vi "Error Lookup.vi"(8 "error in (no error)":errorcluster, 10 "Error code":i32, 11 "VISA resource name":refnum<visa-resource-name>) -> (0 "error out":errorcluster, 2 "Error Message":string, 3 "VISA resource name out":refnum<visa-resource-name>)   [LabVIEW 2012, in "Fluke 8508.lvlib"]
doc: "This utility VI references an instrument error code and returns the corresponding error description message."
uses:
  Fluke 8508.lvlib
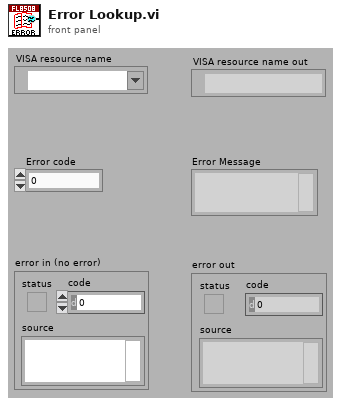
[diagram p1: front panel]
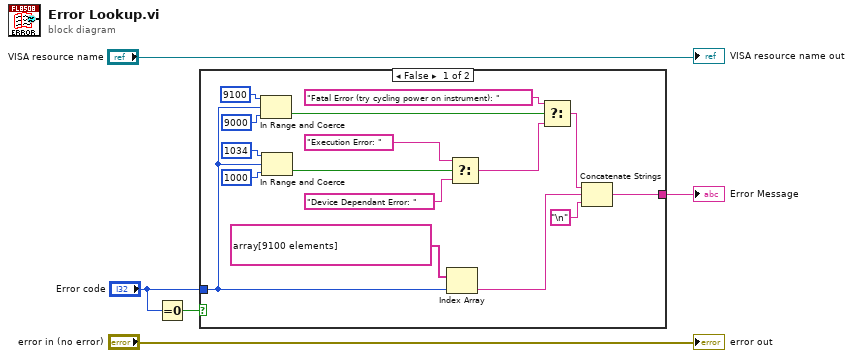
[diagram p0: block diagram]
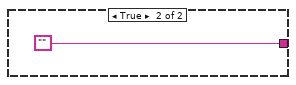
[diagram p2: hidden frame]
diagram:
  n1 = Equal To 0?(x="Error code") -> (x = 0?=w1:bool)
  n2 = case shown="False" w1 {
    tunnel: "Error code" -> [w20 _]
    tunnel: [w6 ""] -> w4
    frame False {
      n3 = In Range and Coerce(upper limit=9100, x=w20, lower limit=9000) -> (In Range?=w17:bool)  [unwired: 1 out]
      n4 = In Range and Coerce(upper limit=1034 ("lower limit"), x=w20, lower limit=1000) -> (In Range?=w16:bool)  [unwired: 1 out]
      n5 = Index Array(array=string[] array[9100 elements], index=w20) -> (element=w8:string)
      n6 = Select(t="Execution Error: ", s=w16, f="Device Dependant Error: ") -> (s? t:f=w11:string)
      n7 = Select(t="Fatal Error (try cycling power on instrument): ", s=w17, f=w11) -> (s? t:f=w9:string)
      n8 = Concatenate Strings(w9, w8, "\n" ("string")) -> (w6:string)
    }
    frame True {
    }
  }
  "Error Message" <- w4
  "error out" <- "error in (no error)"
  "VISA resource name out" <- "VISA resource name"
